vi "QDMH Exit on Run Time.vi"(8 "error in (no error)":errorcluster) -> (0 "error out":errorcluster)   [LabVIEW 2009]
doc: "This VI will exit LabVIEW when called and when the code is running in the run time engine. Should be placed at the end of the main application.\n\nAAL 9/09"
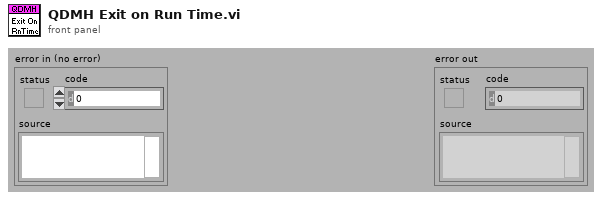
[diagram p1: front panel]
types:
  T1 = enum32{"invalid app kind", "Development System", "Run Time System", "Student Edition", "Embedded LabVIEW", "Evaluation", "Custom"}
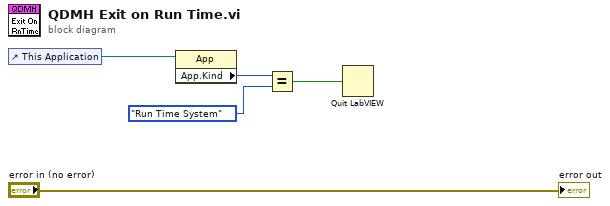
[diagram p0: block diagram]
diagram:
  n1 = control-ref of="This Application"() -> (w5:refnum<vi>)
  n2 = property class="App"(reference=w5) -> ("App.Kind"=w3:T1)  [unwired: 1 in, 2 out]
  n3 = Equal?(x=w3, y=T1."Run Time System" ("Application:Kind")) -> (x = y?=w1:bool)
  n4 = Quit LabVIEW(quit? (T)=w1) -> ()
  "error out" <- "error in (no error)"
